vi "TDT-Check Return Val.vi"(0 "Return Val":i32, 11 "error in (no error)":errorcluster, 13 "source":string="TDT-Interface") -> (15 "error out":errorcluster)   [LabVIEW 2020]
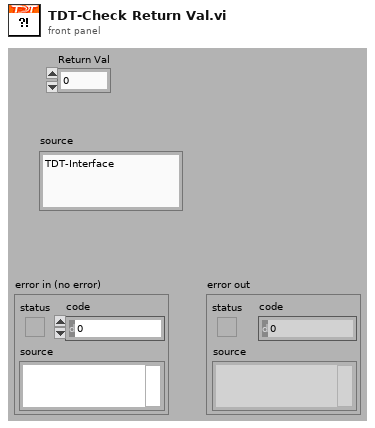
[diagram p1: front panel]
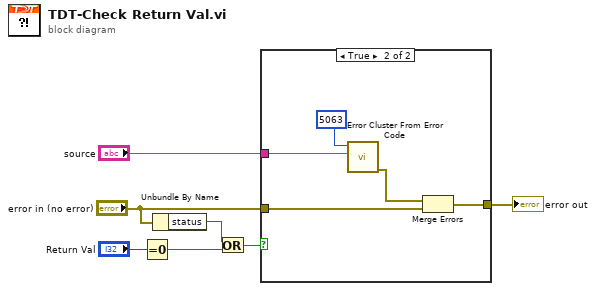
[diagram p0: block diagram]
diagram:
  n1 = Equal To 0?(x="Return Val") -> (x = 0?=w5:bool)
  n2 = Unbundle By Name("error in (no error)") -> ("status"=w6:bool)
  n3 = Or(x=w6, y=w5) -> (x .or. y?=w4:bool)
  n4 = case shown="True" w4 {
    tunnel: "error in (no error)" -> [w8 w13]
    tunnel: "source" -> [_ w11]
    tunnel: [w8 w12] -> w1
    frame False {
    }
    frame True {
      n5 = call <vilib>:"Error Cluster From Error Code.vi"("error message (\"\")"=w11, "error code (0)"=5063 ("code")) -> ("error out"=w10:errorcluster)  [unwired: 7 in]
      n6 = Merge Errors(w10, w13) -> (w12:errorcluster)
    }
  }
  "error out" <- w1
